vi "2.vi"() -> ()   [LabVIEW 2017]
panel:
  out "波形图":dbl[](graph)
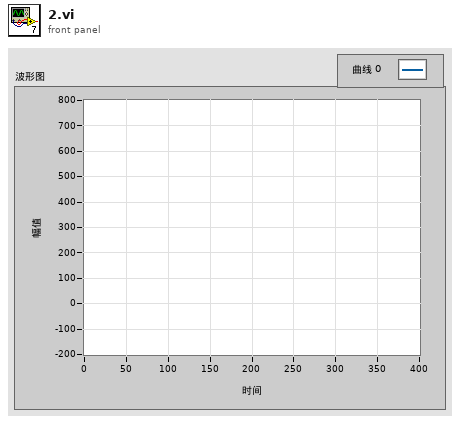
[diagram p1: front panel]
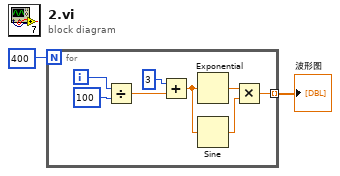
[diagram p0: block diagram]
diagram:
  n1 = for {
    N: 400 -> [_]
    tunnel: [w6] -> w1 mode=indexing
    i -> [w5]
    n2 = Divide(x=w5, y=100) -> (x/y=w3:dbl)
    n3 = Add(x=3, y=w3) -> (x+y=w9:dbl)
    n4 = Exponential(1:w9) -> (0:w8:dbl)
    n5 = Sine(x=w9) -> (sin(x)=w7:dbl)
    n6 = Multiply(x=w8, y=w7) -> (x*y=w6:dbl)
  }
  "波形图" <- w1
